vi "usb set Port Current Limit.vi"(7 "microamps":u32, 8 "error in (no error)":errorcluster, 9 "channel":u8, 10 "result":cluster{"value":i32, "error":i32}, 11 "id":u32) -> (0 "error out":errorcluster, 2 "result out":cluster{"value":i32, "error":i32}, 3 "id out":u32)   [LabVIEW 2014, in "BrainStem2_LabVIEW_Library.lvlib"]
doc: "aLIBEXPORT void __stdcall usb_setPortCurrentLimit ( unsigned int* id, struct Result* result , const unsigned char channel , const unsigned int microamps ) ;"
uses:
  BrainStem2_LabVIEW_Library.lvlib
  BrainStem2_LabVIEW.dll
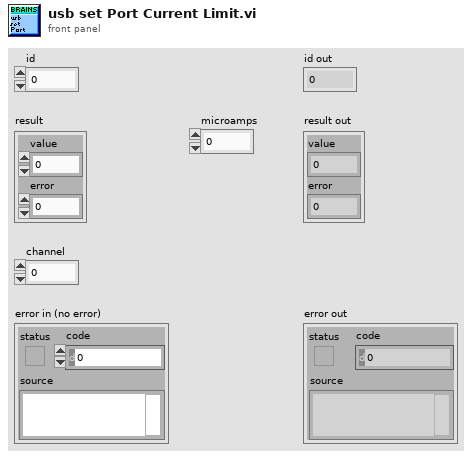
[diagram p1: front panel]
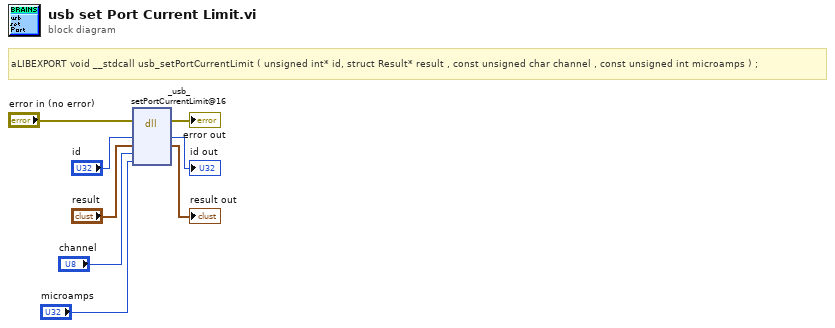
[diagram p0: block diagram]
diagram:
  # "aLIBEXPORT void __stdcall usb_setPortCurrentLimit ( unsigned int* id, struct Result* result , const unsigned char channel , const unsigned int microamps ) ;"
  n1 = dll-call lib="C:/Users/mitch/Documents/development/acroname/software/acroname/aSource/BrainStem2/BrainStem2_LabVIEW/LabVIEW_2014_Distribution/BrainStem2_LabVIEW_w32/BrainStem2_LabVIEW.*" fn="_usb_setPortCurrentLimit@16"(error in="error in (no error)", "id"="id", "result"="result", "channel"="channel", "microamps"="microamps") -> (error out=→"error out":errorcluster, "id"=→"id out":u32, "result"=→"result out":cluster{"value":i32, "error":i32})  [unwired: 5 in, 1 out]
